vi "Button To Toggle Vr3.vi"(1 "InValue":bool) -> (0 "Result":bool)   [LabVIEW 2013]
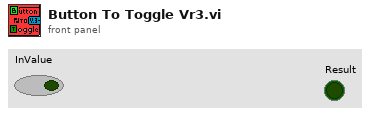
[diagram p1: front panel]
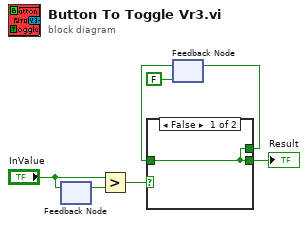
[diagram p0: block diagram]
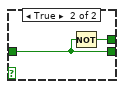
[diagram p2: hidden frame]
diagram:
  n1 = feedback #1() -> (w4:bool)  [unwired: 1 in]
  n2 = feedback-in #1("InValue") -> ()
  n3 = Greater?(x="InValue", y=w4) -> (0:w5:bool)
  n4 = feedback #2(FALSE) -> (w2:bool)
  n5 = case shown="False" w5 {
    tunnel: w2 -> [w8 w9]
    tunnel: [w8 w10] -> w1
    tunnel: [w8 w9] -> w6
    frame False {
    }
    frame True {
      n6 = Not(x=w9) -> (.not. x?=w10:bool)
    }
  }
  "Result" <- w6
  n7 = feedback-in #2(w1) -> ()
